vi "Next Page.vi"(8 "error in (no error)":errorcluster, 11 "HVAC System Model in":refnum<class "HVAC System Model.lvclass">) -> (0 "error out":errorcluster, 3 "HVAC System Model out":refnum<class "HVAC System Model.lvclass">)   [LabVIEW 2013, in "HVAC System Model.lvlib" / "HVAC System Model.lvclass"]
uses:
  HVAC System Model.lvclass
  HVAC System Model.lvclass/HVAC System Model.ctl
  <vilib>/ActorFrameworkMVC/View Observer/View Registry/View Registry.lvclass/View Registry.ctl
  HVAC System Model Messages/Abstract HVAC System Move In Next Msg/Abstract HVAC System Move In Next Msg.lvclass
  <vilib>/ActorFrameworkMVC/View Observer/View Registry/View Registry.lvclass
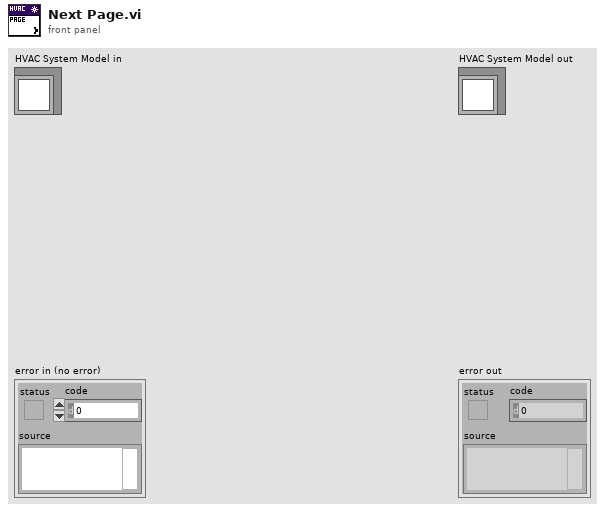
[diagram p1: front panel]
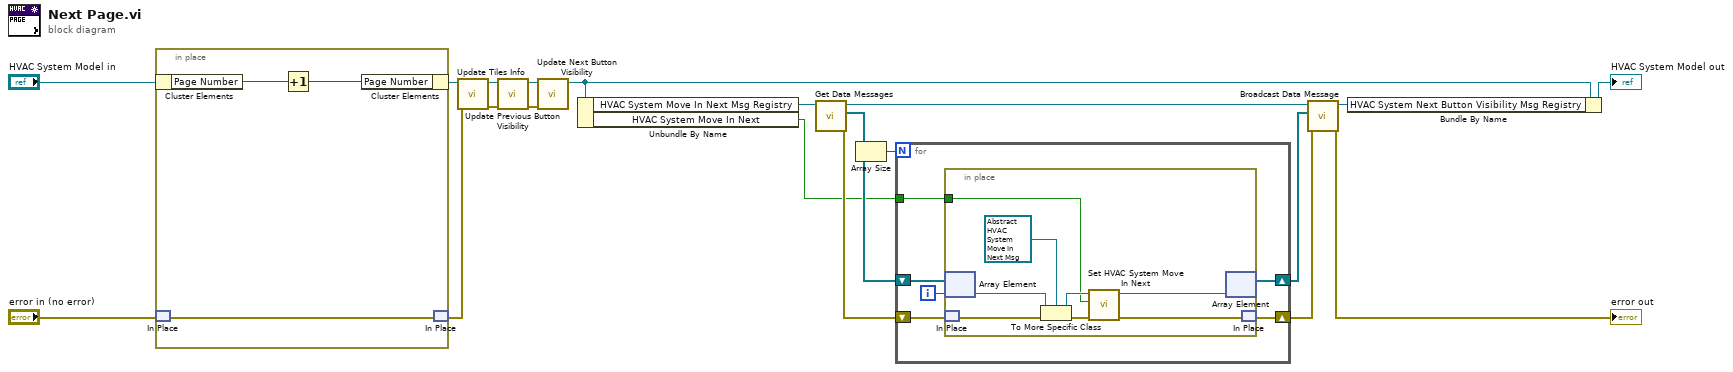
[diagram p0: block diagram]
diagram:
  n1 = in-place {
    n2 = in-place-cluster #1("HVAC System Model in") -> ("Page Number"=w23:i32)
    n3 = in-place-match #2("error in (no error)") -> (w21:errorcluster)
    n4 = Increment(x=w23) -> (x+1=w22:i32)
    n5 = in-place-cluster #1("Page Number"=w22) -> (w13:refnum<class "HVAC System Model.lvclass">)
    n6 = in-place-match #2(w21) -> (w8:errorcluster)
  }
  n7 = call "Update Tiles Info.vi"("error in (no error)"=w8, "HVAC System Model in"=w13) -> ("error out"=w7:errorcluster, "HVAC System Model out"=w12:refnum<class "HVAC System Model.lvclass">)  [unwired: 8 in]
  n8 = call "Update Previous Button Visibility.vi"("error in (no error)"=w7, "HVAC System Model in"=w12) -> ("error out"=w6:errorcluster, "HVAC System Model out"=w11:refnum<class "HVAC System Model.lvclass">)  [unwired: 8 in]
  n9 = call "Update Next Button Visibility.vi"("error in (no error)"=w6, "HVAC System Model in"=w11) -> ("HVAC System Model out"=w5:refnum<class "HVAC System Model.lvclass">)  [unwired: 8 in, 1 out]
  n10 = Unbundle By Name(w5) -> ("HVAC System Move In Next Msg Registry"=w10:refnum<class "View Registry.lvclass">, "HVAC System Move In Next"=w14:bool)
  n11 = call <vilib>:"Get Data Messages.vi"("View Registry in"=w10) -> ("error out"=w18:errorcluster, "Data Messages"=w19:refnum<class "Data Message.lvclass">[], "View Registry out"=w9:refnum<class "View Registry.lvclass">)  [unwired: 8 in]
  n12 = Array Size(array=w19) -> (size(s)=w20:i32)
  n13 = for {
    N: w20 -> [_]
    shift-right: [w28] -> w17
    shift-left: w19 -> [w29]
    shift-right: [w25] -> w16
    shift-left: w18 -> [w27]
    tunnel: w14 -> [w26]
    i -> [w24]
    n14 = in-place {
      in-place-border: w26 -> [w30]
      n15 = in-place-array #3(w29, w24) -> (w35:refnum<class "Data Message.lvclass">)
      n16 = in-place-match #4(w27) -> (w37:errorcluster)
      n17 = To More Specific Class(target class=refnum<class "Abstract HVAC System Move In Next Msg.lvclass"> refnum ("HVAC System Model.lvlib:Abstract HVAC System Move In Next Msg.lvclass"), reference=w35, error in=w37) -> (specific class reference=w31:refnum<class "Abstract HVAC System Move In Next Msg.lvclass">, error out=w34:errorcluster)
      n18 = call "Set HVAC System Move In Next.vi"("error in (no error)"=w34, "HVAC System Move In Next"=w30, "Abstract HVAC System Move In Next Msg in"=w31) -> ("error out"=w33:errorcluster, "Abstract HVAC System Move In Next Msg out"=w32:refnum<class "Abstract HVAC System Move In Next Msg.lvclass">)  [unwired: 7 in]
      n19 = in-place-array #3(w32) -> (w28:refnum<class "Data Message.lvclass">[])  [unwired: 1 out]
      n20 = in-place-match #4(w33) -> (w25:errorcluster)
    }
  }
  n21 = call <vilib>:"Broadcast Data Message.vi"("error in (no error)"=w16, "Data Messages"=w17, "View Registry in"=w9) -> ("error out"=→"error out":errorcluster, "View Registry out"=w15:refnum<class "View Registry.lvclass">)  [unwired: 7 in]
  n22 = Bundle By Name(cluster=w5, "HVAC System Next Button Visibility Msg Registry"=w15) -> (→"HVAC System Model out":refnum<class "HVAC System Model.lvclass">)
